vi "Custom Processing.vi"(0 "tagged llp packets cluster in":T1, 1 "reset":bool, 5 "end of data in":bool[](array[boolean])=[FALSE, FALSE, FALSE, FALSE, FALSE, FALSE, FALSE, FALSE], 9 "input valid":bool[](array[boolean])=[FALSE, FALSE, FALSE, FALSE, FALSE, FALSE, FALSE, FALSE], 12 "ready for output":bool[](array[boolean])=[TRUE, FALSE, FALSE, FALSE, FALSE, FALSE, FALSE, FALSE]) -> (4 "tagged llp packets cluster out":T1, 6 "end of data out":bool[](array[boolean]), 10 "output valid":bool[](array[boolean]), 14 "ready for input":bool[](array[boolean]))   [LabVIEW 2020, in "GettingStarted_Acq_Tap_148X_FPGA.lvlib"]
uses:
  GettingStarted_Acq_Tap_148X_FPGA.lvlib
  Common/Types/Tagged LLP Packets Cluster.ctl
  <instrlib>/FlexRIO/CSI-2/v2/FPGA/Types/Tagged LLP Packet.ctl
  <instrlib>/FlexRIO/CSI-2/v2/FPGA/Types/FPGA LLP Packet Tag.ctl
  <instrlib>/FlexRIO/CSI-2/v2/FPGA/Types/FPGA LLP Packet Timestamp.ctl
  <instrlib>/FlexRIO/CSI-2/v2/FPGA/Types/Timestamp ID.ctl
  <instrlib>/FlexRIO/CSI-2/v2/FPGA/Types/FPGA LLP Packet Size.ctl
  <instrlib>/FlexRIO/CSI-2/v2/FPGA/Types/LLP Packet.ctl
  <instrlib>/FlexRIO/CSI-2/v2/FPGA/Types/LLP Packet Header.ctl
  <instrlib>/FlexRIO/CSI-2/v2/FPGA/Types/LLP Packet Payload.ctl
  <instrlib>/FlexRIO/CSI-2/v2/FPGA/Types/LLP Packet Footer.ctl
  <instrlib>/_niInstr/Basic Elements/v1/FPGA/niInstr Basic Elements v1 FPGA.lvlib
  <instrlib>/FlexRIO/CSI-2/v2/FPGA/NI CSI-2 API FPGA v2.lvlib
  Common/GettingStarted_Common_148X_FPGA.lvlib
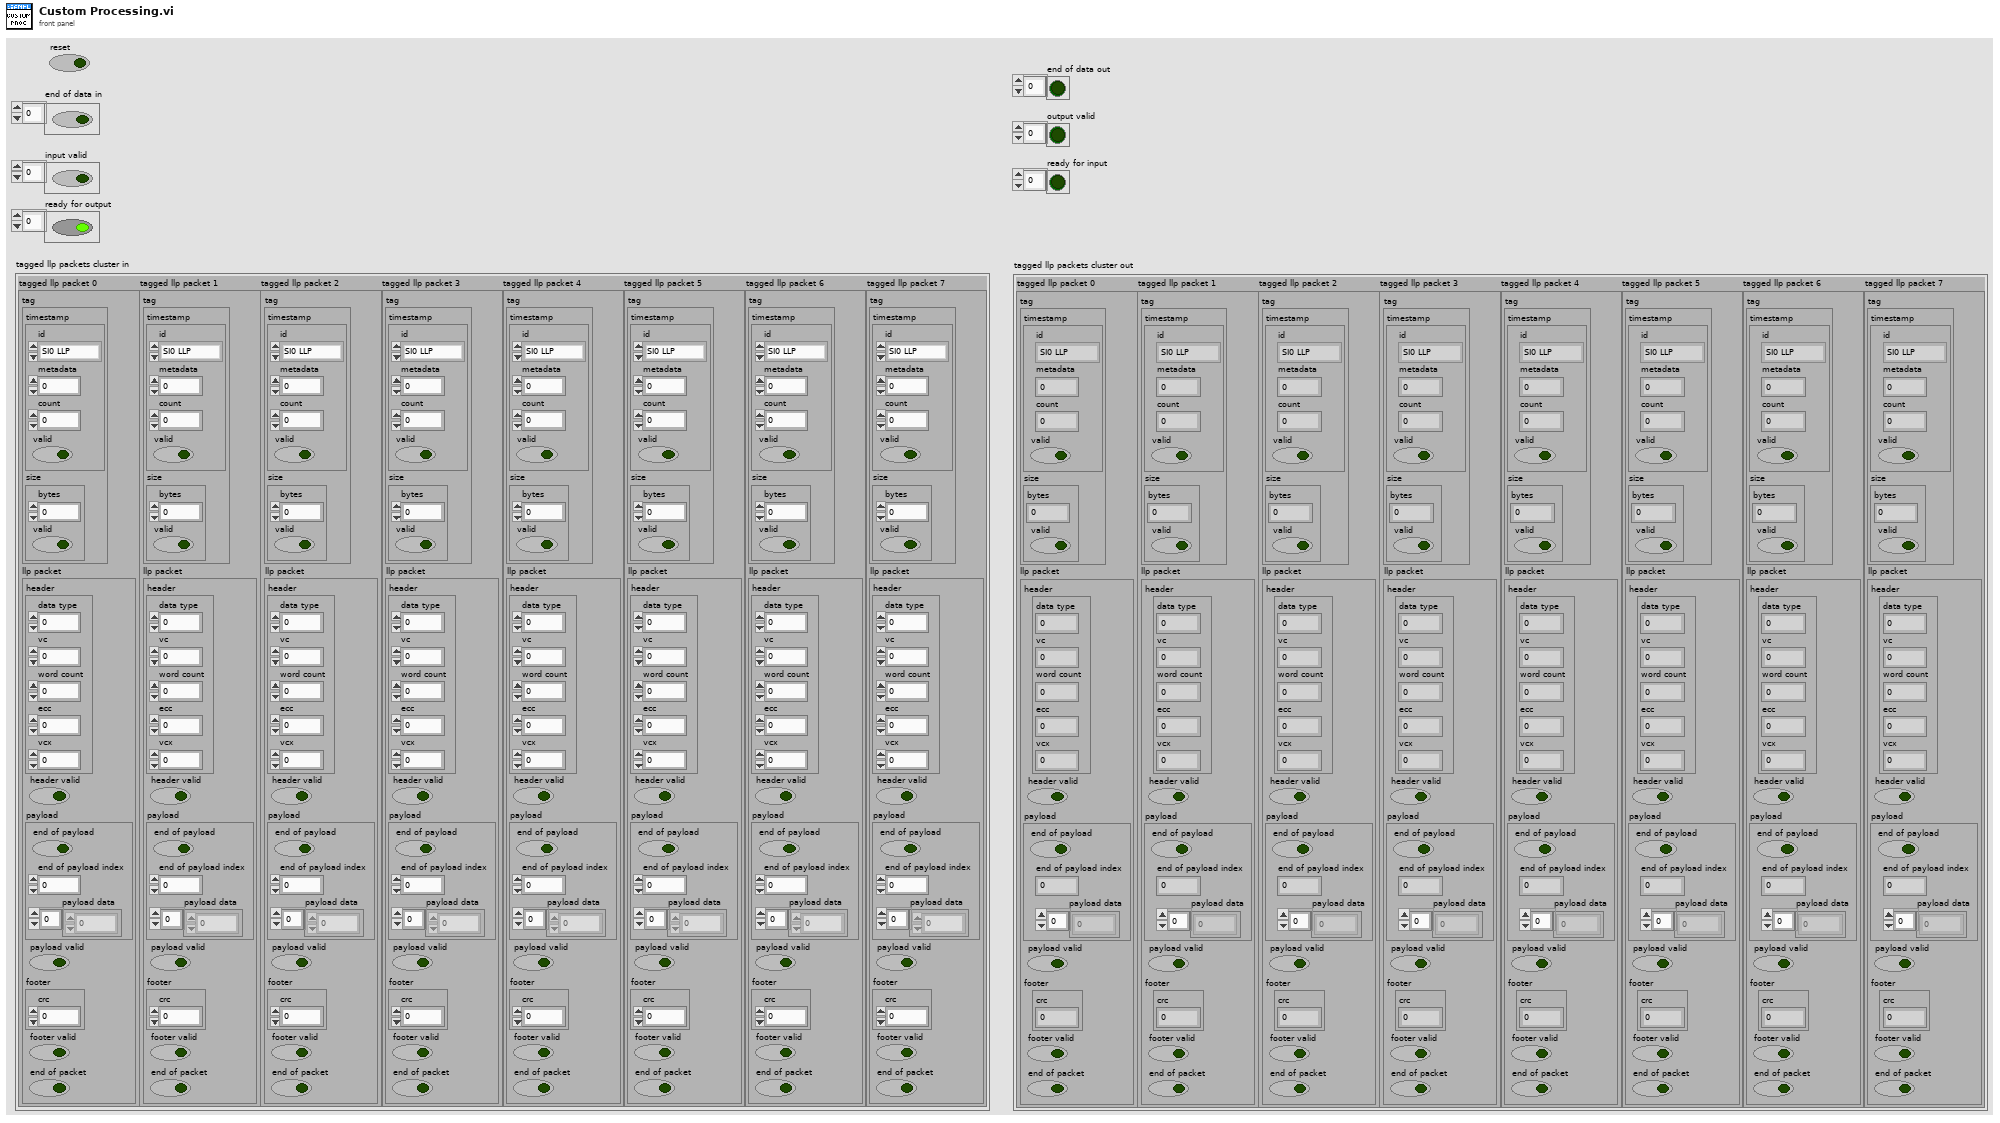
[diagram p1: front panel]
types:
  T1 = typedef "GettingStarted_Common_148X_FPGA.lvlib/Tagged LLP Packets Cluster.ctl" = cluster{"tagged llp packet 0":T2, "tagged llp packet 1":T2, "tagged llp packet 2":T2, "tagged llp packet 3":T2, "tagged llp packet 4":T2, "tagged llp packet 5":T2, "tagged llp packet 6":T2, "tagged llp packet 7":T2}
  T2 = typedef "NI CSI-2 API FPGA v2.lvlib/Tagged LLP Packet.ctl" = cluster{"tag":T3, "llp packet":T7}
  T3 = typedef "NI CSI-2 API FPGA v2.lvlib/FPGA LLP Packet Tag.ctl" = cluster{"timestamp":T4, "size":T6}
  T4 = typedef "NI CSI-2 API FPGA v2.lvlib/FPGA LLP Packet Timestamp.ctl" = cluster{"valid":bool, "count":fxp<+,50,50>, "id":T5, "metadata":u8}
  T5 = typedef "NI CSI-2 API FPGA v2.lvlib/Timestamp ID.ctl" = enum8{"SI0 LLP", "SI1 LLP", "SI2 LLP", "SI3 LLP", "SI4 LLP", "SI5 LLP", "SI6 LLP", "SI7 LLP", "SO0 LLP", "SO1 LLP", "SO2 LLP", "SO3 LLP", "SO4 LLP", "SO5 LLP", "SO6 LLP", "SO7 LLP", "Ser0 GPIO Bank", "Ser1 GPIO Bank", "Ser2 GPIO Bank", "Ser3 GPIO Bank", "Ser4 GPIO Bank", "Ser5 GPIO Bank", "Ser6 GPIO Bank", "Ser7 GPIO Bank", "Des0 GPIO Bank", "Des1 GPIO Bank", "Des2 GPIO Bank", "Des3 GPIO Bank", "Des4 GPIO Bank", "Des5 GPIO Bank", "Des6 GPIO Bank", "Des7 GPIO Bank", "User0", "User1", "User2", "User3", "User4", "User5", "User6", "User7", "User8", "User9", "User10", "User11", "User12", "User13", "User14", "User15", "User16", "User17", "User18", "User19", "User20", "User21", "User22", "User23", "User24", "User25", "User26", "User27", "User28", "User29", "User30", "User31"}
  T6 = typedef "NI CSI-2 API FPGA v2.lvlib/FPGA LLP Packet Size.ctl" = cluster{"bytes":fxp<+,17,17>, "valid":bool}
  T7 = typedef "NI CSI-2 API FPGA v2.lvlib/LLP Packet.ctl" = cluster{"header":T8, "header valid":bool, "payload":T9, "payload valid":bool, "footer":T10, "footer valid":bool, "end of packet":bool}
  T8 = typedef "NI CSI-2 API FPGA v2.lvlib/LLP Packet Header.ctl" = cluster{"word count":u16, "ecc":fxp<+,6,6>, "vcx":fxp<+,2,2>, "data type":fxp<+,6,6>, "vc":fxp<+,2,2>}
  T9 = typedef "NI CSI-2 API FPGA v2.lvlib/LLP Packet Payload.ctl" = cluster{"end of payload":bool, "end of payload index":fxp<+,3,3>, "payload data":u8[]}
  T10 = typedef "NI CSI-2 API FPGA v2.lvlib/LLP Packet Footer.ctl" = cluster{"crc":u16}
  T11 = cluster{"tagged llp packet":T2, "end of data in":bool, "input valid":bool, "ready for output":bool}
  T12 = cluster{"end of data out":bool, "output valid":bool, "ready for input":bool}
  T13 = cluster{"end of data out":bool, "output valid":bool, "ready for input":bool}[]
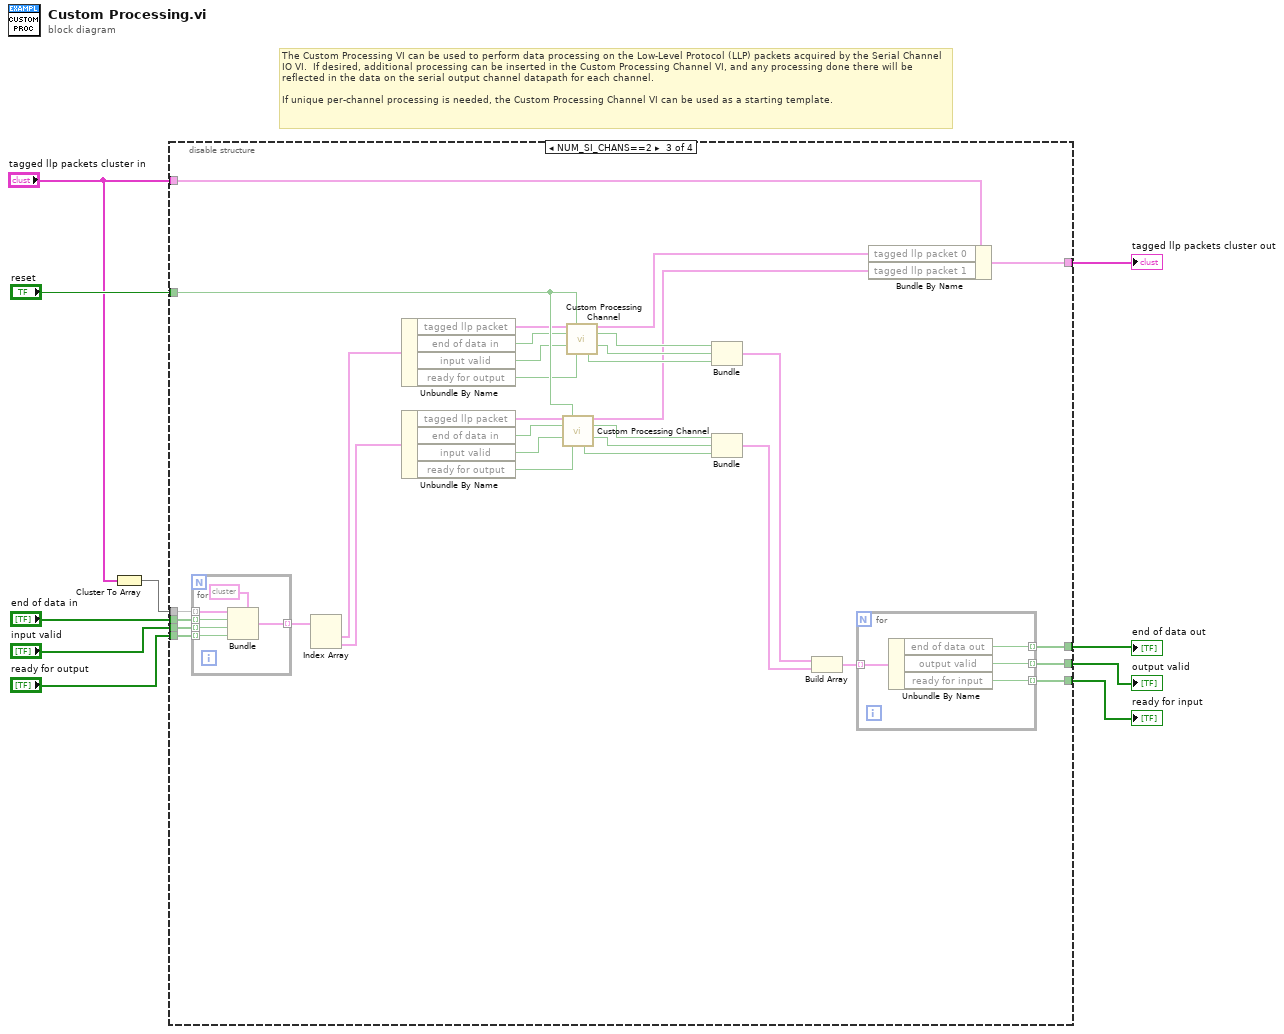
[diagram p0: block diagram]
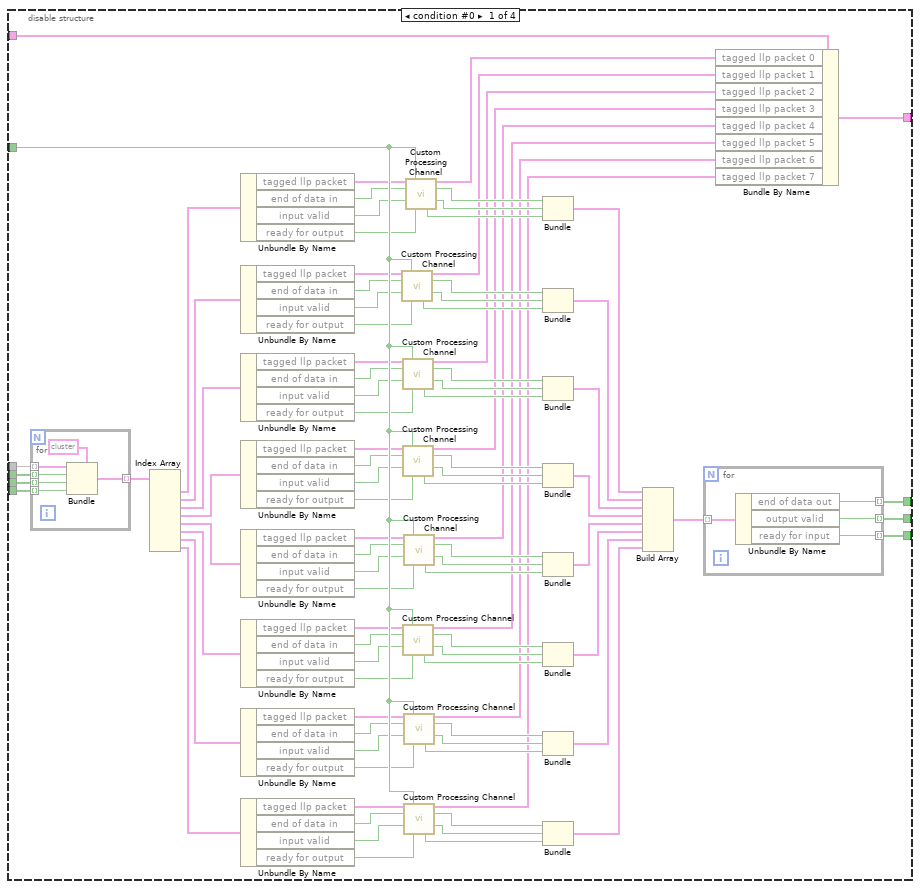
[diagram p2: hidden frame]
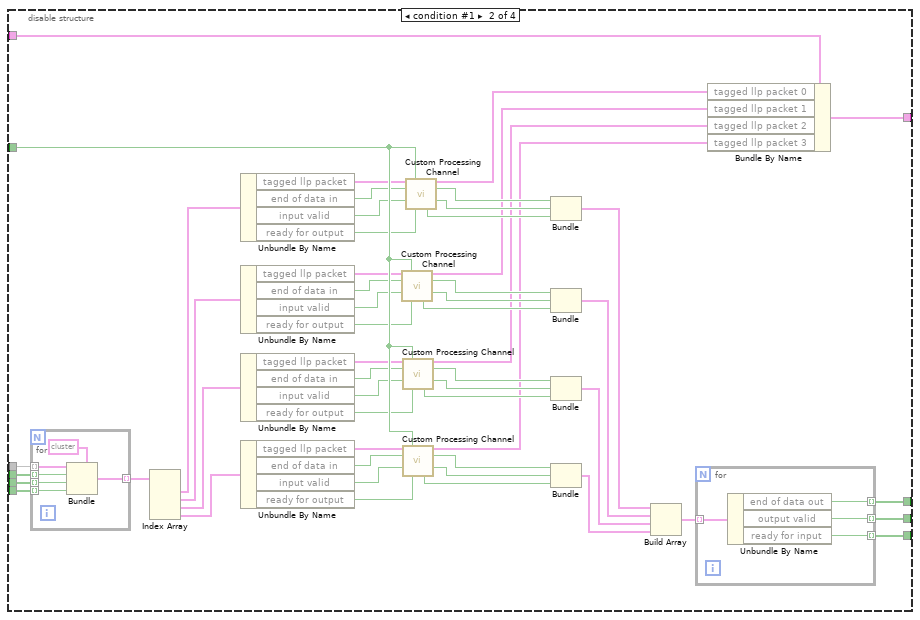
[diagram p3: hidden frame]
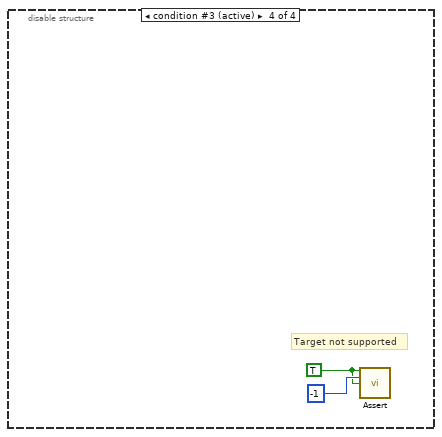
[diagram p4: hidden frame]
diagram:
  # "The Custom Processing VI can be used to perform data processing on the Low-Level Protocol (LLP) packets acquired by the Serial Channel IO VI.  If desired, additional processing can be inserted in the Custom Processing Channel VI, and any processing done there will be reflected in the data on the serial output channel datapath for each channel.\n\nIf unique per-channel processing is needed, the Custom Processing Channel VI can be used as a starting template."
  n1 = Cluster To Array(cluster="tagged llp packets cluster in") -> (array=w2:T2[])
  n2 = disable-structure shown="NUM_SI_CHANS==2" {
    disable-tunnel: "reset" -> [w92 w160 w204 _]
    disable-tunnel: "end of data in" -> [w102 w118 w178 _]
    disable-tunnel: "input valid" -> [w82 w119 w179 _]
    disable-tunnel: "ready for output" -> [w65 w120 w180 _]
    disable-tunnel: [w56 w142 w194 _] -> w5
    disable-tunnel: [w55 w141 w193 _] -> w6
    disable-tunnel: [w30 w128 w186 _] -> w4
    disable-tunnel: [w21 w127 w185 _] -> w3
    disable-tunnel: w2 -> [w20 w121 w181 _]
    disable-tunnel: "tagged llp packets cluster in" -> [w11 w113 w175 _]
    frame condition #0 {
      n3 = for {
        tunnel: w102 -> [w107] mode=indexing
        tunnel: [w108] -> w101 mode=indexing
        tunnel: w82 -> [w106] mode=indexing
        tunnel: w65 -> [w105] mode=indexing
        tunnel: w20 -> [w103] mode=indexing
        n4 = Bundle(cluster=T11 {"tagged llp packet"={"tag"={"timestamp"={"valid"=FALSE, "count"=0.0, "id"=enum."SI0 LLP", "metadata"=0}, "size"={"bytes"=0.0, "valid"=FALSE}}, "llp packet"={"header"={"word count"=0, "ecc"=0.0, "vcx"=0.0, "data type"=0.0, "vc"=0.0}, "header valid"=FALSE, "payload"={"end of payload"=FALSE, "end of payload index"=0.0, "payload data"=[]}, "payload valid"=FALSE, "footer"={"crc"=0}, "footer valid"=FALSE, "end of packet"=FALSE}}, "end of data in"=FALSE, "input valid"=FALSE, "ready for output"=FALSE}, "tagged llp packet"=w103, "end of data in"=w107, "input valid"=w106, "ready for output"=w105) -> (w108:T11)
      }
      n5 = Index Array(array=w101) -> (element #1=w100:T11, element #2=w97:T11, element #3=w96:T11, element #4=w94:T11, element #5=w93:T11, element #6=w95:T11, element #7=w98:T11, element #8=w99:T11)  [unwired: 8 in]
      n6 = Unbundle By Name(w100) -> ("tagged llp packet"=w19:T2, "end of data in"=w80:bool, "input valid"=w81:bool, "ready for output"=w64:bool)
      n7 = Unbundle By Name(w97) -> ("tagged llp packet"=w18:T2, "end of data in"=w79:bool, "input valid"=w78:bool, "ready for output"=w63:bool)
      n8 = Unbundle By Name(w96) -> ("tagged llp packet"=w17:T2, "end of data in"=w77:bool, "input valid"=w76:bool, "ready for output"=w62:bool)
      n9 = Unbundle By Name(w94) -> ("tagged llp packet"=w16:T2, "end of data in"=w75:bool, "input valid"=w74:bool, "ready for output"=w61:bool)
      n10 = Unbundle By Name(w93) -> ("tagged llp packet"=w12:T2, "end of data in"=w73:bool, "input valid"=w72:bool, "ready for output"=w60:bool)
      n11 = Unbundle By Name(w95) -> ("tagged llp packet"=w13:T2, "end of data in"=w71:bool, "input valid"=w70:bool, "ready for output"=w59:bool)
      n12 = Unbundle By Name(w98) -> ("tagged llp packet"=w14:T2, "end of data in"=w69:bool, "input valid"=w68:bool, "ready for output"=w58:bool)
      n13 = Unbundle By Name(w99) -> ("tagged llp packet"=w15:T2, "end of data in"=w67:bool, "input valid"=w66:bool, "ready for output"=w57:bool)
      n14 = call "Custom Processing Channel.vi"("tagged llp packet in"=w18, "reset"=w92, "end of data in"=w79, "input valid"=w78, "ready for output"=w63) -> ("tagged llp packet out"=w23:T2, "end of data out"=w51:bool, "output valid"=w50:bool, "ready for input"=w49:bool)  [unwired: 7 in]
      n15 = call "Custom Processing Channel.vi"("tagged llp packet in"=w17, "reset"=w92, "end of data in"=w77, "input valid"=w76, "ready for output"=w62) -> ("tagged llp packet out"=w24:T2, "end of data out"=w42:bool, "output valid"=w41:bool, "ready for input"=w48:bool)  [unwired: 7 in]
      n16 = call "Custom Processing Channel.vi"("tagged llp packet in"=w16, "reset"=w92, "end of data in"=w75, "input valid"=w74, "ready for output"=w61) -> ("tagged llp packet out"=w25:T2, "end of data out"=w40:bool, "output valid"=w39:bool, "ready for input"=w47:bool)  [unwired: 7 in]
      n17 = call "Custom Processing Channel.vi"("tagged llp packet in"=w13, "reset"=w92, "end of data in"=w71, "input valid"=w70, "ready for output"=w59) -> ("tagged llp packet out"=w27:T2, "end of data out"=w36:bool, "output valid"=w35:bool, "ready for input"=w45:bool)  [unwired: 7 in]
      n18 = call "Custom Processing Channel.vi"("tagged llp packet in"=w12, "reset"=w92, "end of data in"=w73, "input valid"=w72, "ready for output"=w60) -> ("tagged llp packet out"=w26:T2, "end of data out"=w38:bool, "output valid"=w37:bool, "ready for input"=w46:bool)  [unwired: 7 in]
      n19 = call "Custom Processing Channel.vi"("tagged llp packet in"=w14, "reset"=w92, "end of data in"=w69, "input valid"=w68, "ready for output"=w58) -> ("tagged llp packet out"=w28:T2, "end of data out"=w34:bool, "output valid"=w33:bool, "ready for input"=w44:bool)  [unwired: 7 in]
      n20 = call "Custom Processing Channel.vi"("tagged llp packet in"=w15, "reset"=w92, "end of data in"=w67, "input valid"=w66, "ready for output"=w57) -> ("tagged llp packet out"=w29:T2, "end of data out"=w32:bool, "output valid"=w31:bool, "ready for input"=w43:bool)  [unwired: 7 in]
      n21 = call "Custom Processing Channel.vi"("tagged llp packet in"=w19, "reset"=w92, "end of data in"=w80, "input valid"=w81, "ready for output"=w64) -> ("tagged llp packet out"=w22:T2, "end of data out"=w52:bool, "output valid"=w53:bool, "ready for input"=w54:bool)  [unwired: 7 in]
      n22 = Bundle("end of data out"=w52, "output valid"=w53, "ready for input"=w54) -> (w89:T12)  [unwired: 1 in]
      n23 = Bundle("end of data out"=w51, "output valid"=w50, "ready for input"=w49) -> (w86:T12)  [unwired: 1 in]
      n24 = Bundle("end of data out"=w42, "output valid"=w41, "ready for input"=w48) -> (w85:T12)  [unwired: 1 in]
      n25 = Bundle("end of data out"=w40, "output valid"=w39, "ready for input"=w47) -> (w91:T12)  [unwired: 1 in]
      n26 = Bundle("end of data out"=w38, "output valid"=w37, "ready for input"=w46) -> (w90:T12)  [unwired: 1 in]
      n27 = Bundle("end of data out"=w36, "output valid"=w35, "ready for input"=w45) -> (w84:T12)  [unwired: 1 in]
      n28 = Bundle("end of data out"=w34, "output valid"=w33, "ready for input"=w44) -> (w87:T12)  [unwired: 1 in]
      n29 = Bundle("end of data out"=w32, "output valid"=w31, "ready for input"=w43) -> (w88:T12)  [unwired: 1 in]
      n30 = Build Array(w89, w86, w85, w91, w90, w84, w87, w88) -> (w83:T13)
      n31 = for {
        tunnel: w83 -> [w112] mode=indexing
        tunnel: [w111] -> w56 mode=indexing
        tunnel: [w110] -> w55 mode=indexing
        tunnel: [w109] -> w30 mode=indexing
        n32 = Unbundle By Name(w112) -> ("end of data out"=w111:bool, "output valid"=w110:bool, "ready for input"=w109:bool)
      }
      n33 = Bundle By Name(cluster=w11, "tagged llp packet 0"=w22, "tagged llp packet 1"=w23, "tagged llp packet 2"=w24, "tagged llp packet 3"=w25, "tagged llp packet 4"=w26, "tagged llp packet 5"=w27, "tagged llp packet 6"=w28, "tagged llp packet 7"=w29) -> (w21:T1)
    }
    frame condition #1 {
      n34 = for {
        tunnel: w118 -> [w169] mode=indexing
        tunnel: [w170] -> w122 mode=indexing
        tunnel: w119 -> [w168] mode=indexing
        tunnel: w120 -> [w167] mode=indexing
        tunnel: w121 -> [w165] mode=indexing
        n35 = Bundle(cluster=T11 {"tagged llp packet"={"tag"={"timestamp"={"valid"=FALSE, "count"=0.0, "id"=enum."SI0 LLP", "metadata"=0}, "size"={"bytes"=0.0, "valid"=FALSE}}, "llp packet"={"header"={"word count"=0, "ecc"=0.0, "vcx"=0.0, "data type"=0.0, "vc"=0.0}, "header valid"=FALSE, "payload"={"end of payload"=FALSE, "end of payload index"=0.0, "payload data"=[]}, "payload valid"=FALSE, "footer"={"crc"=0}, "footer valid"=FALSE, "end of packet"=FALSE}}, "end of data in"=FALSE, "input valid"=FALSE, "ready for output"=FALSE}, "tagged llp packet"=w165, "end of data in"=w169, "input valid"=w168, "ready for output"=w167) -> (w170:T11)
      }
      n36 = Index Array(array=w122) -> (element #1=w164:T11, element #2=w163:T11, element #3=w162:T11, element #4=w161:T11)  [unwired: 4 in]
      n37 = Unbundle By Name(w164) -> ("tagged llp packet"=w117:T2, "end of data in"=w153:bool, "input valid"=w154:bool, "ready for output"=w146:bool)
      n38 = Unbundle By Name(w163) -> ("tagged llp packet"=w116:T2, "end of data in"=w152:bool, "input valid"=w151:bool, "ready for output"=w145:bool)
      n39 = Unbundle By Name(w162) -> ("tagged llp packet"=w115:T2, "end of data in"=w150:bool, "input valid"=w149:bool, "ready for output"=w144:bool)
      n40 = Unbundle By Name(w161) -> ("tagged llp packet"=w114:T2, "end of data in"=w148:bool, "input valid"=w147:bool, "ready for output"=w143:bool)
      n41 = call "Custom Processing Channel.vi"("tagged llp packet in"=w116, "reset"=w160, "end of data in"=w152, "input valid"=w151, "ready for output"=w145) -> ("tagged llp packet out"=w124:T2, "end of data out"=w137:bool, "output valid"=w136:bool, "ready for input"=w135:bool)  [unwired: 7 in]
      n42 = call "Custom Processing Channel.vi"("tagged llp packet in"=w115, "reset"=w160, "end of data in"=w150, "input valid"=w149, "ready for output"=w144) -> ("tagged llp packet out"=w125:T2, "end of data out"=w132:bool, "output valid"=w131:bool, "ready for input"=w134:bool)  [unwired: 7 in]
      n43 = call "Custom Processing Channel.vi"("tagged llp packet in"=w114, "reset"=w160, "end of data in"=w148, "input valid"=w147, "ready for output"=w143) -> ("tagged llp packet out"=w126:T2, "end of data out"=w130:bool, "output valid"=w129:bool, "ready for input"=w133:bool)  [unwired: 7 in]
      n44 = call "Custom Processing Channel.vi"("tagged llp packet in"=w117, "reset"=w160, "end of data in"=w153, "input valid"=w154, "ready for output"=w146) -> ("tagged llp packet out"=w123:T2, "end of data out"=w138:bool, "output valid"=w139:bool, "ready for input"=w140:bool)  [unwired: 7 in]
      n45 = Bundle("end of data out"=w138, "output valid"=w139, "ready for input"=w140) -> (w158:T12)  [unwired: 1 in]
      n46 = Bundle("end of data out"=w137, "output valid"=w136, "ready for input"=w135) -> (w157:T12)  [unwired: 1 in]
      n47 = Bundle("end of data out"=w132, "output valid"=w131, "ready for input"=w134) -> (w156:T12)  [unwired: 1 in]
      n48 = Bundle("end of data out"=w130, "output valid"=w129, "ready for input"=w133) -> (w159:T12)  [unwired: 1 in]
      n49 = Build Array(w158, w157, w156, w159) -> (w155:T13)
      n50 = for {
        tunnel: w155 -> [w174] mode=indexing
        tunnel: [w173] -> w142 mode=indexing
        tunnel: [w172] -> w141 mode=indexing
        tunnel: [w171] -> w128 mode=indexing
        n51 = Unbundle By Name(w174) -> ("end of data out"=w173:bool, "output valid"=w172:bool, "ready for input"=w171:bool)
      }
      n52 = Bundle By Name(cluster=w113, "tagged llp packet 0"=w123, "tagged llp packet 1"=w124, "tagged llp packet 2"=w125, "tagged llp packet 3"=w126) -> (w127:T1)
    }
    frame condition #2 {
      n53 = for {
        tunnel: w178 -> [w211] mode=indexing
        tunnel: [w212] -> w182 mode=indexing
        tunnel: w179 -> [w210] mode=indexing
        tunnel: w180 -> [w209] mode=indexing
        tunnel: w181 -> [w207] mode=indexing
        n54 = Bundle(cluster=T11 {"tagged llp packet"={"tag"={"timestamp"={"valid"=FALSE, "count"=0.0, "id"=enum."SI0 LLP", "metadata"=0}, "size"={"bytes"=0.0, "valid"=FALSE}}, "llp packet"={"header"={"word count"=0, "ecc"=0.0, "vcx"=0.0, "data type"=0.0, "vc"=0.0}, "header valid"=FALSE, "payload"={"end of payload"=FALSE, "end of payload index"=0.0, "payload data"=[]}, "payload valid"=FALSE, "footer"={"crc"=0}, "footer valid"=FALSE, "end of packet"=FALSE}}, "end of data in"=FALSE, "input valid"=FALSE, "ready for output"=FALSE}, "tagged llp packet"=w207, "end of data in"=w211, "input valid"=w210, "ready for output"=w209) -> (w212:T11)
      }
      n55 = Index Array(array=w182) -> (element #1=w206:T11, element #2=w205:T11)  [unwired: 2 in]
      n56 = Unbundle By Name(w206) -> ("tagged llp packet"=w177:T2, "end of data in"=w199:bool, "input valid"=w200:bool, "ready for output"=w196:bool)
      n57 = Unbundle By Name(w205) -> ("tagged llp packet"=w176:T2, "end of data in"=w198:bool, "input valid"=w197:bool, "ready for output"=w195:bool)
      n58 = call "Custom Processing Channel.vi"("tagged llp packet in"=w176, "reset"=w204, "end of data in"=w198, "input valid"=w197, "ready for output"=w195) -> ("tagged llp packet out"=w184:T2, "end of data out"=w189:bool, "output valid"=w188:bool, "ready for input"=w187:bool)  [unwired: 7 in]
      n59 = call "Custom Processing Channel.vi"("tagged llp packet in"=w177, "reset"=w204, "end of data in"=w199, "input valid"=w200, "ready for output"=w196) -> ("tagged llp packet out"=w183:T2, "end of data out"=w190:bool, "output valid"=w191:bool, "ready for input"=w192:bool)  [unwired: 7 in]
      n60 = Bundle("end of data out"=w190, "output valid"=w191, "ready for input"=w192) -> (w203:T12)  [unwired: 1 in]
      n61 = Bundle("end of data out"=w189, "output valid"=w188, "ready for input"=w187) -> (w202:T12)  [unwired: 1 in]
      n62 = Build Array(w203, w202) -> (w201:T13)
      n63 = for {
        tunnel: w201 -> [w216] mode=indexing
        tunnel: [w215] -> w194 mode=indexing
        tunnel: [w214] -> w193 mode=indexing
        tunnel: [w213] -> w186 mode=indexing
        n64 = Unbundle By Name(w216) -> ("end of data out"=w215:bool, "output valid"=w214:bool, "ready for input"=w213:bool)
      }
      n65 = Bundle By Name(cluster=w175, "tagged llp packet 0"=w183, "tagged llp packet 1"=w184) -> (w185:T1)
    }
    frame condition #3 (active) {
      w217 = TRUE ("assert")
      # "Target not supported"
      n66 = call <instrlib>:"Assert.vi"("assert"=w217, "error code"=-1, "enable show error"=w217) -> ()  [unwired: 13 in]
    }
  }
  "output valid" <- w6
  "ready for input" <- w4
  "end of data out" <- w5
  "tagged llp packets cluster out" <- w3
